vi "Write count.vi"(8 "error in (no error)":errorcluster, 10 "count":i32, 11 "Relay in":refnum<class "Relay.lvclass">) -> (0 "error out":errorcluster, 3 "Relay out":refnum<class "Relay.lvclass">)   [LabVIEW 2016, in "SLSC Switch.lvlib" / "Relay.lvclass"]
uses:
  Relay.lvclass
  Relay.lvclass/Relay.ctl
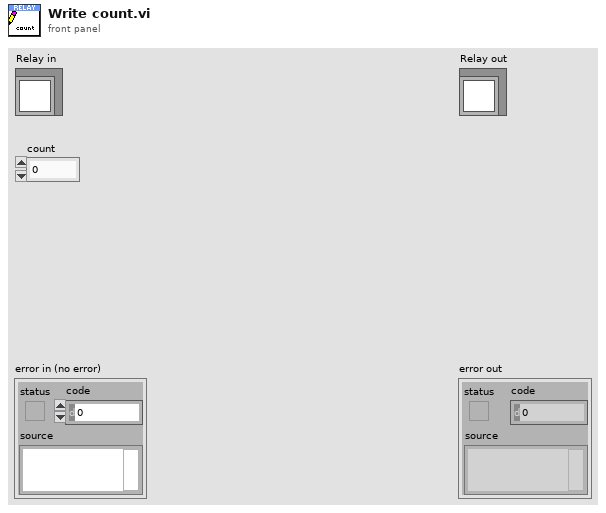
[diagram p1: front panel]
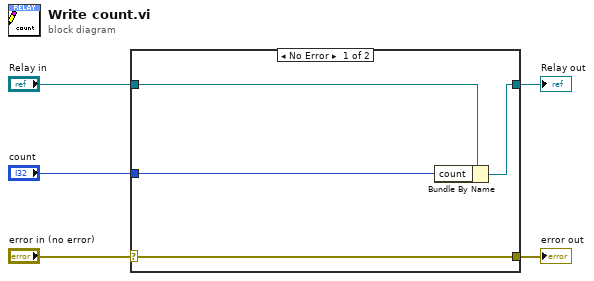
[diagram p0: block diagram]
diagram:
  n1 = case shown="No Error" "error in (no error)" {
    selector: "error in (no error)" -> [w9 w10]
    tunnel: [w9 w10] -> w4
    tunnel: [w7 w11] -> w2
    tunnel: "Relay in" -> [w8 w11]
    tunnel: "count" -> [w6 _]
    frame No Error {
      n2 = Bundle By Name(cluster=w8, "count"=w6) -> (w7:refnum<class "Relay.lvclass">)
    }
    frame Error {
    }
  }
  "error out" <- w4
  "Relay out" <- w2
